vi "baseStation-single.vi"() -> ()   [LabVIEW 2012]
uses:
  <vilib>/Instr/_visa.llb/VISA Configure Serial Port (Instr).vi
panel:
  out "Thermometer":dbl(slide) scale=0.0..100.0
  out "Relative Humidity":dbl(graph)
  out "Temperature":dbl(graph)
  out "ATM Pressure":dbl(graph)
  out "Magnetic Field":cluster{dbl, dbl, dbl}(graph)
  out "Gyroscope":cluster{dbl, dbl, dbl}(graph)
  out "Accelerometer":cluster{dbl, dbl, dbl}(graph)
  out "error out 2":errorcluster
  in  "Stop Data":bool caption="Blank Button"
  in  "Start Data":bool caption="Blank Button"
  in  "Change Address":bool
  out "Humidity":dbl
  out "Temperature":dbl
  out "Pressure":dbl
  out "Magnetometer":dbl[](array[numeric])
  out "Gyro":dbl[](array[numeric])
  out "Acceleration":dbl[](array[numeric])
  in  "Calibrate":bool caption="Blank Button"
  out "radio ack":bool
  in  "Stop Button":bool
  out "Cal Constants":u8[](array[numeric])
  in  "Radio Address":dbl
  in  "Com port":refnum<visa-resource-name>
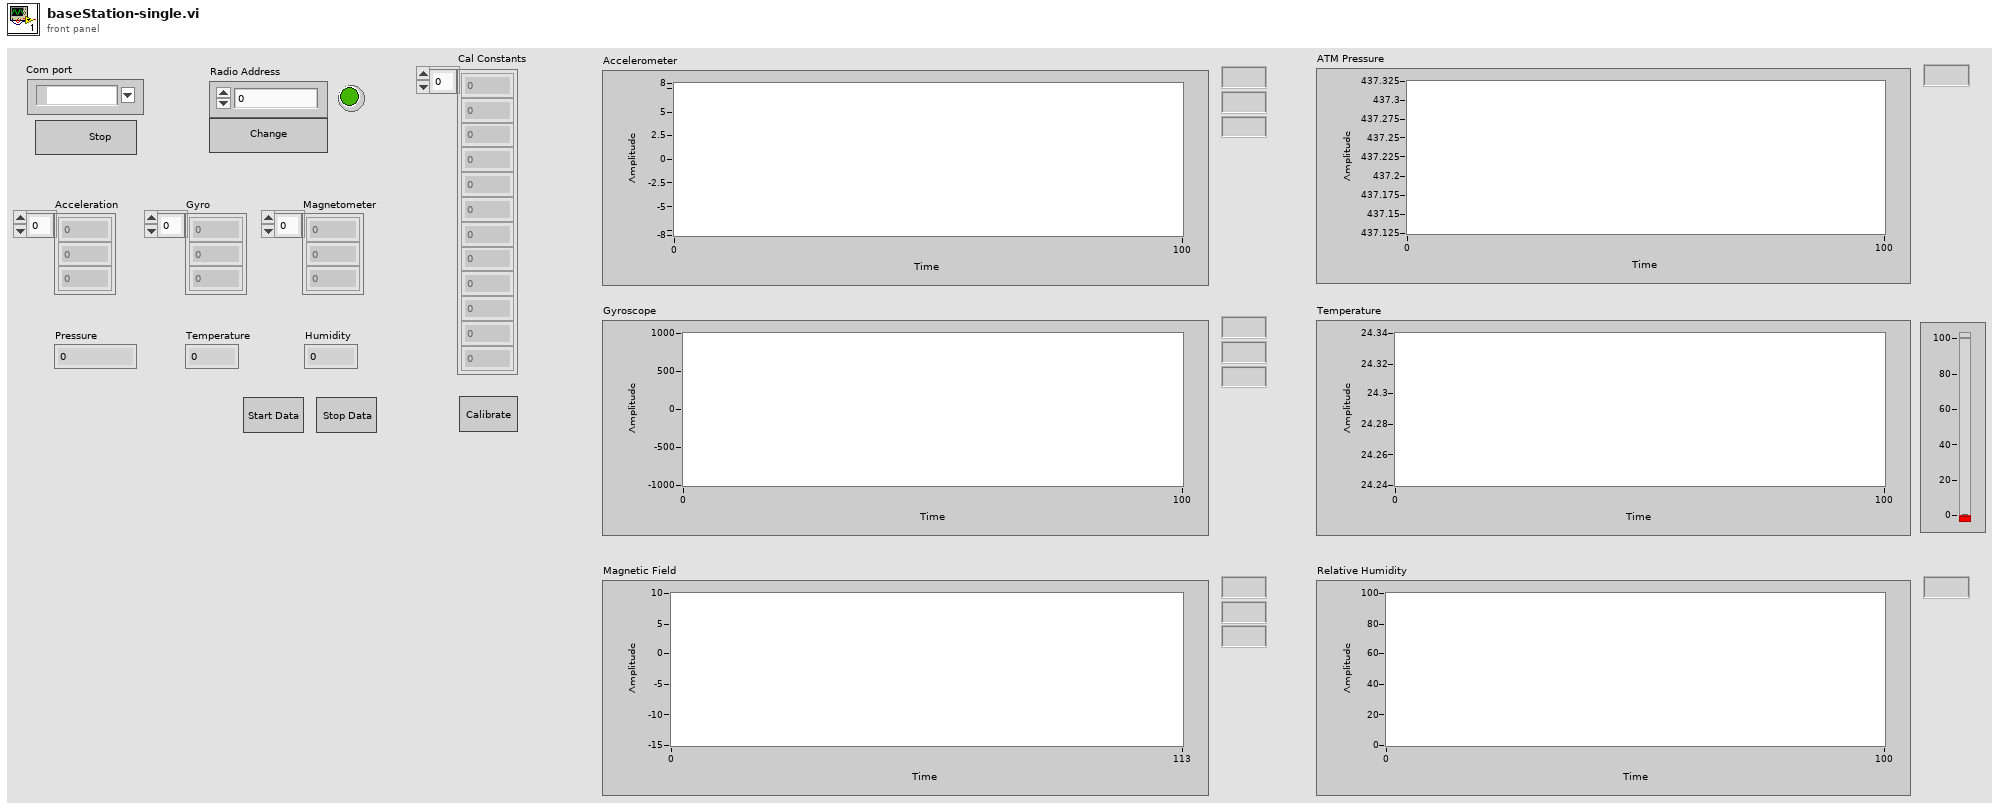
[diagram p1: front panel]
types:
  T1 = cluster{"Acceleration":dbl[], "Gyro":dbl[], "Magnetometer":dbl[], "Temperature":dbl, "Pressure":dbl, "Humidity":dbl}
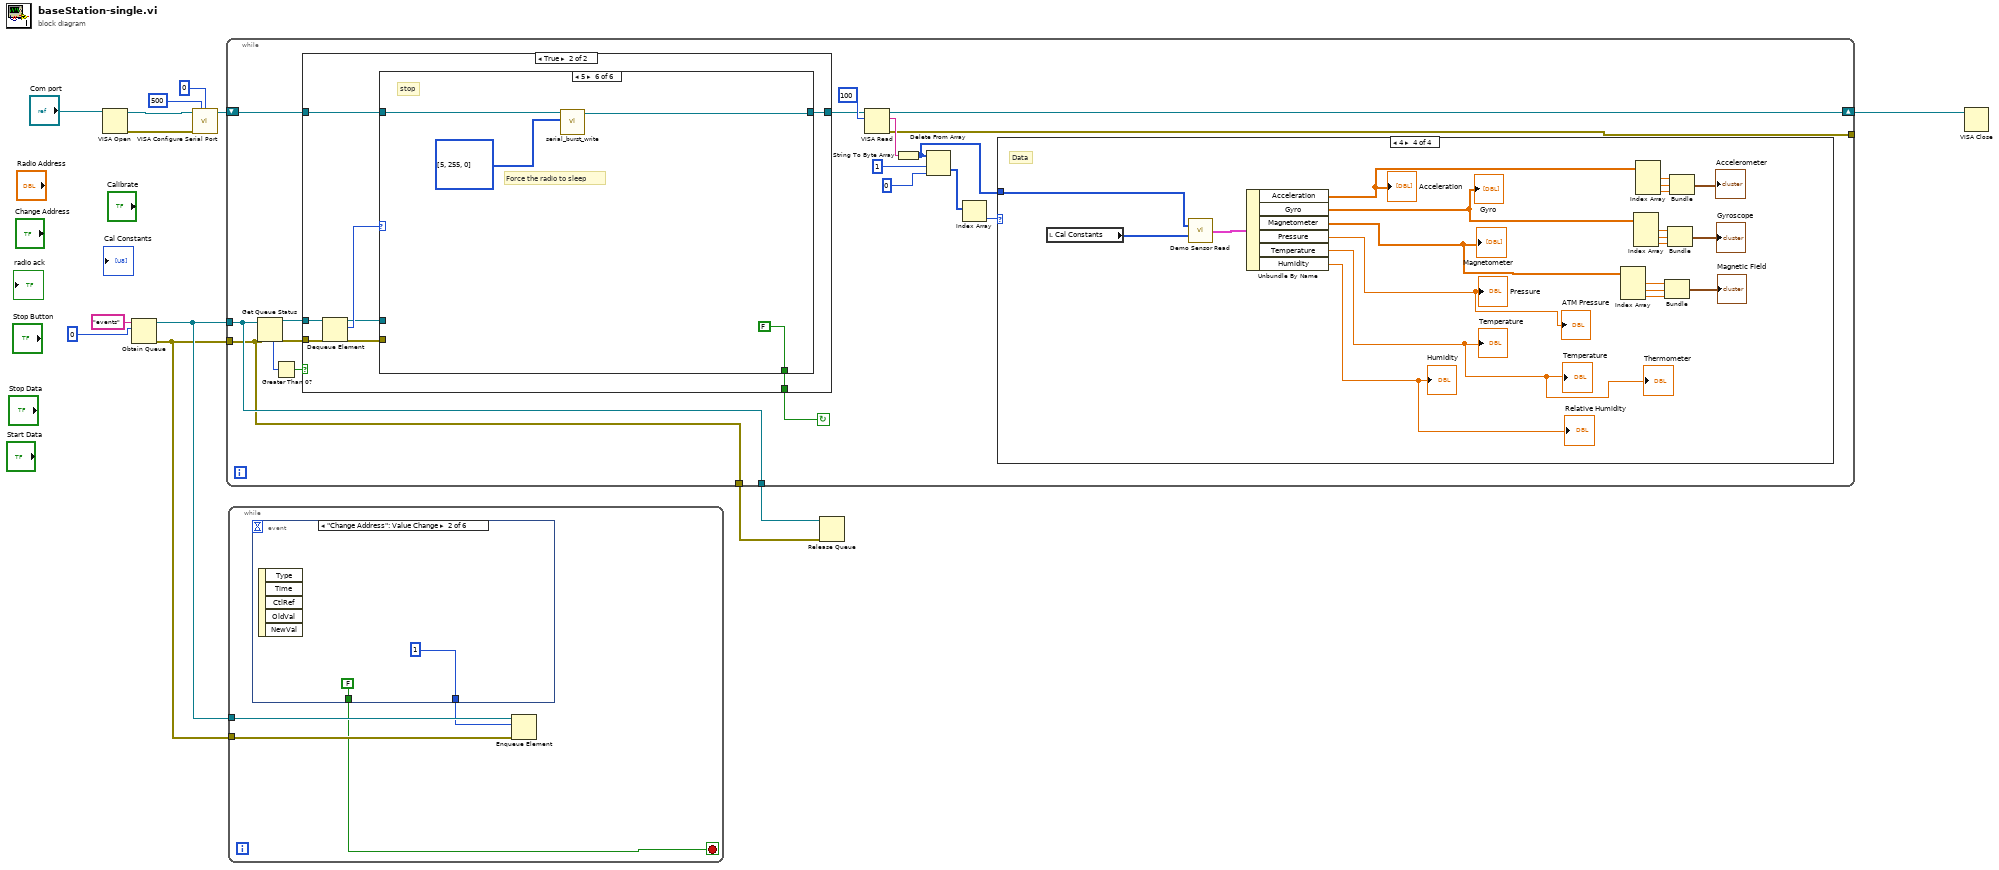
[diagram p0: block diagram]
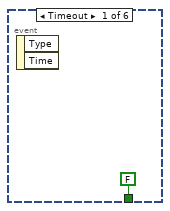
[diagram p2: hidden frame]
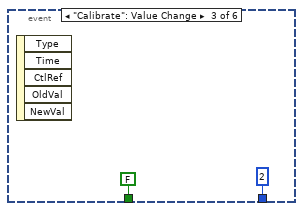
[diagram p3: hidden frame]
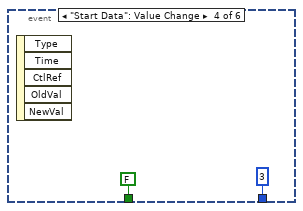
[diagram p4: hidden frame]
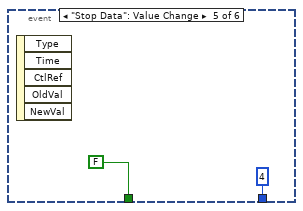
[diagram p5: hidden frame]
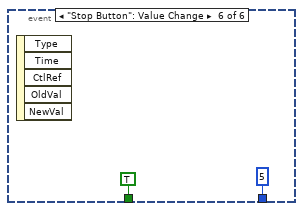
[diagram p6: hidden frame]
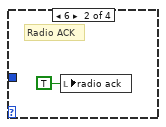
[diagram p8: hidden frame]
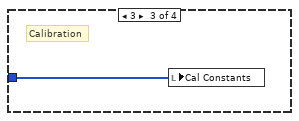
[diagram p9: hidden frame]
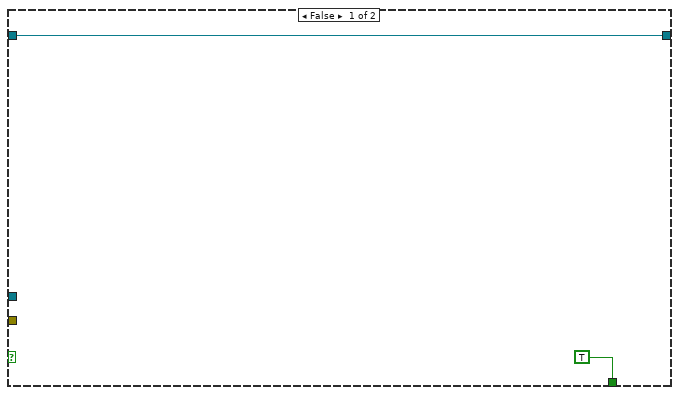
[diagram p10: hidden frame]
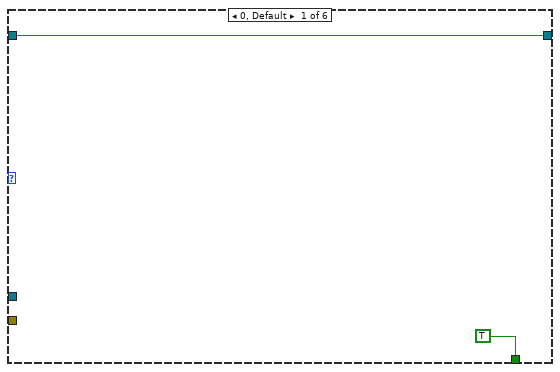
[diagram p11: hidden frame]
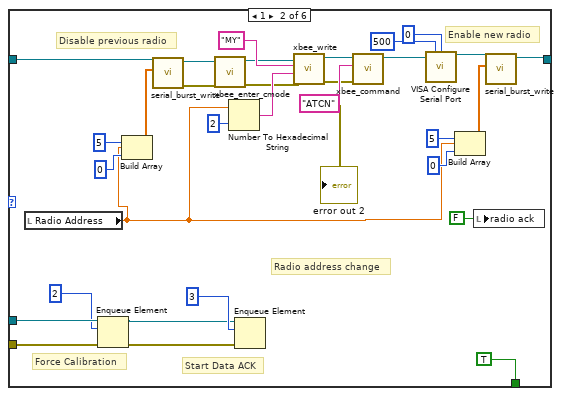
[diagram p12: hidden frame]
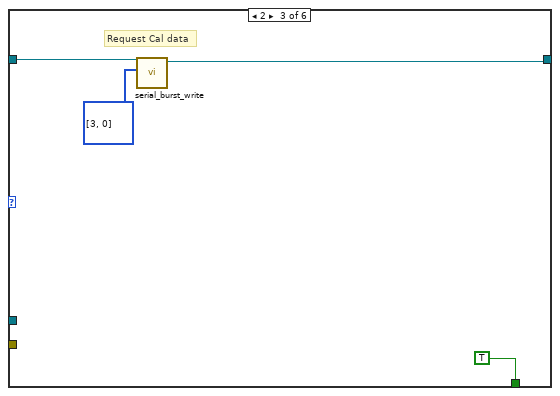
[diagram p13: hidden frame]
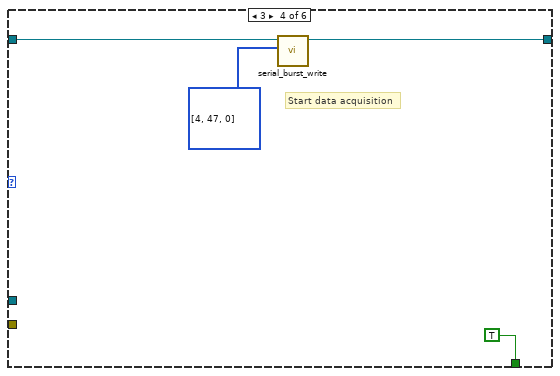
[diagram p14: hidden frame]
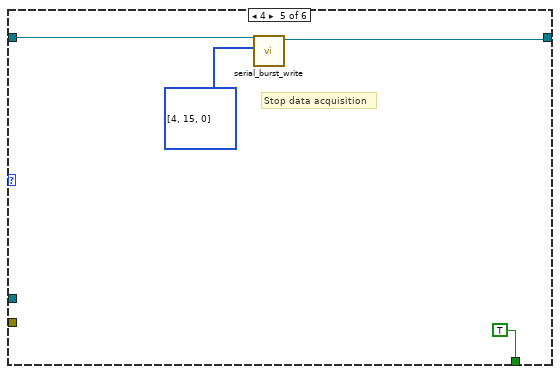
[diagram p15: hidden frame]
diagram:
  n1 = VISA Open(VISA resource name="Com port") -> (VISA resource name=w4:refnum<visa-resource-name>, error out=w5:errorcluster)  [unwired: 4 in]
  n2 = Obtain Queue(name (unnamed)="events", element data type=0) -> (queue out=w10:refnum<queue>, error out=w9:errorcluster)  [unwired: 3 in, 1 out]
  n3 = call-poly "VISA Configure Serial Port"("VISA resource name"=w4, "timeout (10sec)"=u32 500, "termination char\n(0xA = '\\n' = LF)"=u8 0 ("termination char\n(0xA = '\\n' = LF)"), "error in (no error)"=w5) -> ("VISA resource name out"=w6:refnum<visa-resource-name>)  [unwired: 10 in, 1 out]
  n4 = while {
    tunnel: w10 -> [w17]
    tunnel: w9 -> [w16]
    shift-right: [w27] -> w8
    shift-left: w6 -> [w31]
    tunnel: [w17] -> w2
    tunnel: [w16] -> w1
    tunnel: [w14] -> _
    stop <- w20 continue-if-true
    n5 = Get Queue Status(queue=w17, error in (no error)=w16) -> (queue out=w22:refnum<queue>, error out=w21:errorcluster, # elements in queue=w18:i32)  [unwired: 1 in, 5 out]
    n6 = Greater Than 0?(x=w18) -> (x > 0?=w19:bool)
    n7 = case shown="True" w19 {
      tunnel: w31 -> [w56 w61]
      tunnel: [w56 w60] -> w29
      tunnel: w22 -> [_ w64]
      tunnel: w21 -> [_ w63]
      tunnel: [TRUE ("radio ack") w57] -> w20
      frame False {
      }
      frame True {
        n8 = Dequeue Element(queue=w64, error in (no error)=w63) -> (queue out=w59:refnum<queue>, element=w62:i32, error out=w58:errorcluster)  [unwired: 1 in, 1 out]
        n9 = case shown="5" w62 {
          tunnel: w61 -> [w66 w84 w101 w104 w109 w113]
          tunnel: [w66 w88 w100 w105 w108 w112] -> w60
          tunnel: w59 -> [_ w81 _ _ _ _]
          tunnel: w58 -> [_ w80 _ _ _ _]
          tunnel: [TRUE ("radio ack") TRUE ("radio ack") TRUE ("radio ack") TRUE ("radio ack") TRUE ("radio ack") FALSE ("radio ack")] -> w57
          frame 0, Default {
          }
          frame 1 {
            # "Start Data ACK"
            # "Force Calibration"
            # "Enable new radio"
            # "Disable previous radio"
            # "Radio address change"
            n10 = local read "Radio Address"() -> (w82:dbl)
            n11 = Enqueue Element(queue=w81, element=2, error in (no error)=w80) -> (queue out=w77:refnum<queue>, error out=w76:errorcluster)  [unwired: 1 in, 1 out]
            n12 = Build Array(u16 5 ("input string"), w82, 0 ("input string")) -> (w87:dbl[])
            n13 = call "serial_burst_write.vi"("Byte array"=w87, "VISA resource name"=w84) -> ("error out"=w70:errorcluster, "VISA resource name out"=w83:refnum<visa-resource-name>)  [unwired: 8 in]
            n14 = call "xbee_enter_cmode.vi"("error in (no error)"=w70, "COM in"=w83) -> ("error out"=w69:errorcluster, "COM out"=w96:refnum<visa-resource-name>)  [unwired: 8 in]
            n15 = Number To Hexadecimal String(1:i16 2 ("width (-)"), 2:w82) -> (0:w93:string)
            n16 = Enqueue Element(queue=w77, element=3, error in (no error)=w76) -> ()  [unwired: 1 in, 3 out]
            n17 = call "xbee_write.vi"("error in"=w69, "value"=w93, "command"="MY", "com in"=w96) -> ("error out"=w68:errorcluster, "com out"=w94:refnum<visa-resource-name>)  [unwired: 6 in]
            n18 = call "xbee_command.vi"("error in (no error)"=w68, "command"="ATCN", "COM in"=w94) -> ("error out"=→"error out 2":errorcluster, "COM out"=w72:refnum<visa-resource-name>)  [unwired: 6 in, 1 out]
            n19 = call-poly "VISA Configure Serial Port"("VISA resource name"=w72, "timeout (10sec)"=u32 500, "termination char\n(0xA = '\\n' = LF)"=u8 0 ("termination char\n(0xA = '\\n' = LF)")) -> ("VISA resource name out"=w71:refnum<visa-resource-name>)  [unwired: 11 in, 1 out]
            n20 = Build Array(u16 5 ("input string"), w82, 0 ("input string")) -> (w91:dbl[])
            n21 = local write "radio ack"(FALSE ("radio ack")) -> ()
            n22 = call "serial_burst_write.vi"("Byte array"=w91, "VISA resource name"=w71) -> ("VISA resource name out"=w88:refnum<visa-resource-name>)  [unwired: 8 in, 1 out]
          }
          frame 2 {
            # "Request Cal data"
            n23 = call "serial_burst_write.vi"("Byte array"=u16[] [3, 0], "VISA resource name"=w101) -> ("VISA resource name out"=w100:refnum<visa-resource-name>)  [unwired: 8 in, 1 out]
          }
          frame 3 {
            # "Start data acquisition"
            n24 = call "serial_burst_write.vi"("Byte array"=u16[] [4, 47, 0], "VISA resource name"=w104) -> ("VISA resource name out"=w105:refnum<visa-resource-name>)  [unwired: 8 in, 1 out]
          }
          frame 4 {
            # "Stop data acquisition"
            n25 = call "serial_burst_write.vi"("Byte array"=u16[] [4, 15, 0], "VISA resource name"=w109) -> ("VISA resource name out"=w108:refnum<visa-resource-name>)  [unwired: 8 in, 1 out]
          }
          frame 5 {
            # "Force the radio to sleep"
            # "stop"
            n26 = call "serial_burst_write.vi"("Byte array"=u16[] [5, 255, 0], "VISA resource name"=w113) -> ("VISA resource name out"=w112:refnum<visa-resource-name>)  [unwired: 8 in, 1 out]
          }
        }
      }
    }
    n27 = VISA Read(VISA resource name=w29, byte count=u32 100) -> (VISA resource name out=w27:refnum<visa-resource-name>, read buffer=w28:string, error out=w14:errorcluster)  [unwired: 1 in, 1 out]
    n28 = String To Byte Array(string=w28) -> (unsigned byte array=w15:u8[])
    n29 = Delete From Array(array=w15, length=1, index=0) -> (deleted portion=w23:u8[])  [unwired: 1 out]
    n30 = Index Array(array=w23) -> (element=w24:u8)  [unwired: 1 in]
    n31 = case shown="4" w24 {
      tunnel: w15 -> [_ _ w33 w53]
      frame 0, Default {
      }
      frame 6 {
        # "Radio ACK"
        n32 = local write "radio ack"(TRUE ("radio ack")) -> ()
      }
      frame 3 {
        # "Calibration"
        n33 = local write "Cal Constants"(w33) -> ()
      }
      frame 4 {
        # "Data"
        n34 = local read "Cal Constants"() -> (w52:u8[])
        n35 = call "Demo Sensor Read.vi"("baro cal"=w52, "Byte array"=w53) -> ("sensor output"=w54:T1)
        n36 = Unbundle By Name(w54) -> ("Acceleration"=w47:dbl[], "Gyro"=w43:dbl[], "Magnetometer"=w37:dbl[], "Pressure"=→"Pressure" →"ATM Pressure":dbl, "Temperature"=→"Temperature" →"Temperature" →"Thermometer":dbl, "Humidity"=→"Humidity" →"Relative Humidity":dbl)
        "Acceleration" <- w47
        "Gyro" <- w43
        "Magnetometer" <- w37
        n37 = Index Array(array=w37) -> (element #1=w40:dbl, element #2=w39:dbl, element #3=w38:dbl)  [unwired: 3 in]
        n38 = Index Array(array=w43) -> (element #1=w41:dbl, element #2=w46:dbl, element #3=w45:dbl)  [unwired: 3 in]
        n39 = Index Array(array=w47) -> (element #1=w51:dbl, element #2=w50:dbl, element #3=w49:dbl)  [unwired: 3 in]
        n40 = Bundle(w40, w39, w38) -> (→"Magnetic Field":cluster{dbl, dbl, dbl})  [unwired: 1 in]
        n41 = Bundle(w41, w46, w45) -> (→"Gyroscope":cluster{dbl, dbl, dbl})  [unwired: 1 in]
        n42 = Bundle(w51, w50, w49) -> (→"Accelerometer":cluster{dbl, dbl, dbl})  [unwired: 1 in]
      }
    }
  }
  n43 = while {
    tunnel: w10 -> [w118]
    tunnel: w9 -> [w117]
    stop <- w115 stop-if-true
    n44 = event shown="[1] \"Change Address\": Value Change" {
      selector: _ -> [_ _ _ _ _ _]
      dyn-events: _ -> [_ _ _ _ _ _]
      timeout: _ -> [_ _ _ _ _ _]
      tunnel: [_ 1 2 3 4 5] -> w116
      tunnel: [FALSE ("NewVal") FALSE ("NewVal") FALSE ("NewVal") FALSE ("NewVal") FALSE TRUE ("NewVal")] -> w115
      event Timeout {
        n45 = event-data() -> ()  [unwired: 1 in, 2 out]
      }
      event "Change Address": Value Change {
        n46 = event-data() -> ()  [unwired: 1 in, 5 out]
      }
      event "Calibrate": Value Change {
        n47 = event-data() -> ()  [unwired: 1 in, 5 out]
      }
      event "Start Data": Value Change {
        n48 = event-data() -> ()  [unwired: 1 in, 5 out]
      }
      event "Stop Data": Value Change {
        n49 = event-data() -> ()  [unwired: 1 in, 5 out]
      }
      event "Stop Button": Value Change {
        n50 = event-data() -> ()  [unwired: 1 in, 5 out]
      }
    }
    n51 = Enqueue Element(queue=w118, element=w116, error in (no error)=w117) -> ()  [unwired: 1 in, 3 out]
  }
  n52 = Release Queue(queue=w2, error in (no error)=w1) -> ()  [unwired: 1 in, 3 out]
  n53 = VISA Close(VISA resource name=w8) -> ()  [unwired: 1 in, 1 out]
